vi "iTacho_Find Complete Frame-teardown.vi"(6 "Leftover Bytes":string, 7 "test case ID":string, 9 "Found New Frame":bool, 10 "Actual Frame":string, 11 "Expected Frame":string) -> (3 "result":bool)   [LabVIEW 2018]
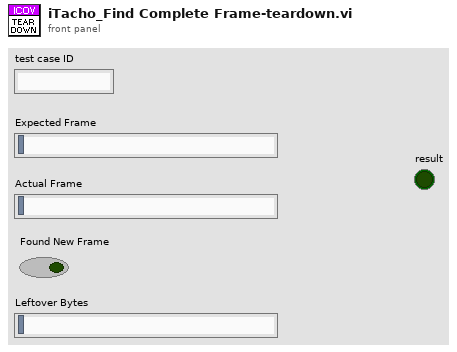
[diagram p1: front panel]
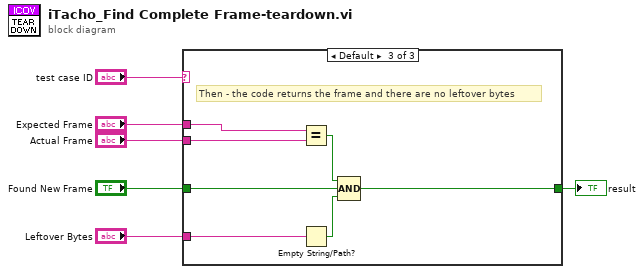
[diagram p0: block diagram]
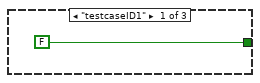
[diagram p2: hidden frame]
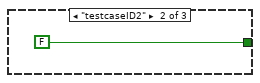
[diagram p3: hidden frame]
diagram:
  n1 = case shown="Default" "test case ID" {
    tunnel: [FALSE FALSE w9] -> w5
    tunnel: "Expected Frame" -> [_ _ w13]
    tunnel: "Actual Frame" -> [_ _ w12]
    tunnel: "Found New Frame" -> [_ _ w11]
    tunnel: "Leftover Bytes" -> [_ _ w10]
    frame "testcaseID1" {
    }
    frame "testcaseID2" {
    }
    frame Default {
      # "Then - the code returns the frame and there are no leftover bytes"
      n2 = Equal?(x=w13, y=w12) -> (x = y?=w14:bool)
      n3 = Empty String/Path?(string/path=w10) -> (empty?=w15:bool)
      n4 = Compound Arithmetic op=AND(w14, w11, w15) -> (w9:bool)
    }
  }
  "result" <- w5
